vi "Open_TestStand_WorkOrders.vi"(8 "error in (no error)":errorcluster, 11 "URL":string="https://epcpower.odoo.com/web#view_type=kanban&model=mrp.workorder&action=554&active_id=3&menu_id=122") -> (0 "error out":errorcluster)   [LabVIEW 2022 SP3]
uses:
  <vilib>/Platform/browser.llb/Open URL in Default Browser (string).vi
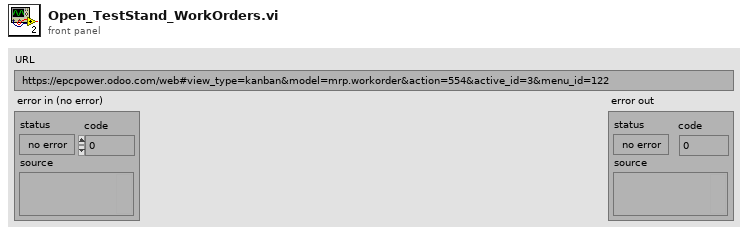
[diagram p1: front panel]
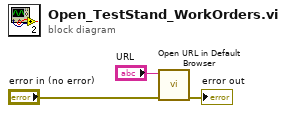
[diagram p0: block diagram]
diagram:
  n1 = call-poly <vilib>:"Open URL in Default Browser.vi"("error in (no error)"="error in (no error)", "URL"="URL") -> ("error out"=→"error out":errorcluster)  [unwired: 4 in, 1 out]
